vi "MQTT_Read_Subscribed_Topics.vi"(8 "error in (no error)":errorcluster) -> (0 "error out":errorcluster)   [LabVIEW 2020, in "MQTT_Functions.lvlib"]
doc: "A basic example that reads topics that the client subcribed to. \n\n© 2015 - daq.io, LLC - Peter Adelhardt"
uses:
  MQTT_Functions.lvlib
  Controls/QoS.ctl
  Controls/Connect_Flags.ctl
  Controls/Retain_Flag.ctl
  Controls/DUP_Flag.ctl
  Controls/User_Info.ctl
  Controls/Connection_Return_Codes.ctl
panel:
  out "Connection Status":T1=enum."Connection refused: not authorized"
  in  "Exit":bool
  in  "MQTT Broker":cluster{"address (IP)":string, "port":u16}={"address (IP)"="172.16.0.250", "port"=1883}
  out "Message IDs":u16[](array[numeric]) format="%x"
  out "Topics":string[](array[string])
  out "Messages":string[](array[string])
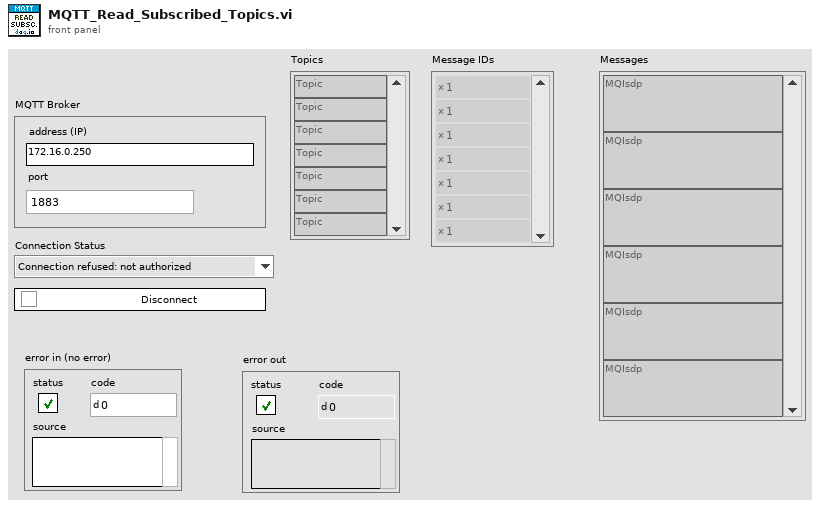
[diagram p1: front panel]
types:
  T1 = typedef "MQTT_Functions.lvlib/Connection_Return_Codes.ctl" = enum16{"Connection accepted", "Connection refused: unacceptable protocol version", "Connection refused: identifier rejected", "Connection refused: Server unavailable", "Connection refused: bad user name or password", "Connection refused: not authorized"}
  T2 = typedef "MQTT_Functions.lvlib/User_Info.ctl" = cluster{"User Name":string, "Password":string}
  T3 = typedef "MQTT_Functions.lvlib/QoS.ctl" = enum8{"At most once", "At least once", "Exactly once", "Reserved"}
  T4 = typedef "MQTT_Functions.lvlib/DUP_Flag.ctl" = bool
  T5 = typedef "MQTT_Functions.lvlib/Retain_Flag.ctl" = bool
  T6 = cluster{"QoS":T3, "DUP":T4, "Retain":T5, "Keep Alive (sec)":u16}
  T7 = typedef "MQTT_Functions.lvlib/Connect_Flags.ctl" = cluster{"user name":bool, "password":bool, "will retain":bool, "will flag":bool, "clean session":bool, "reserved":bool, "will QoS":T3}
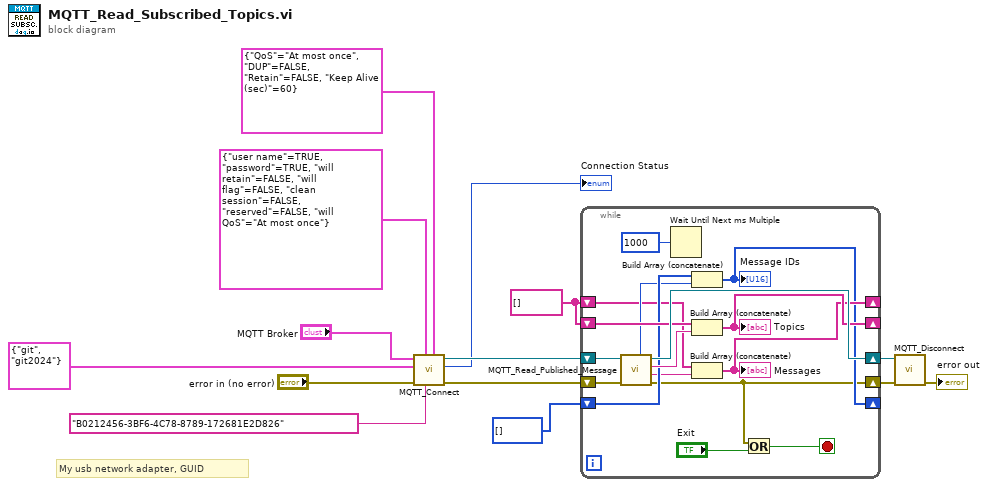
[diagram p0: block diagram]
diagram:
  w7 = string[] []
  # "My usb network adapter, GUID"
  n1 = call "MQTT_Connect.vi"("Connect Meta"=T6 {"QoS"=enum."At most once", "DUP"=FALSE, "Retain"=FALSE, "Keep Alive (sec)"=60}, "Client ID"="B0212456-3BF6-4C78-8789-172681E2D826", "Connect Flags"=T7 {"user name"=TRUE, "password"=TRUE, "will retain"=FALSE, "will flag"=FALSE, "clean session"=FALSE, "reserved"=FALSE, "will QoS"=enum."At most once"}, "error in (no error)"="error in (no error)", "User Info"=T2 {"User Name"="git", "Password"="git2024"}, "MQTT Broker"="MQTT Broker") -> ("error out"=w2:errorcluster, "Connection Status"=→"Connection Status":T1, "connection ID out"=w4:refnum<k5>)  [unwired: 3 in]
  n2 = while {
    shift-right: [w15] -> w9
    shift-left: w2 -> [w27]
    shift-right: [w17] -> _
    shift-left: u16[] [] -> [w23]
    shift-right: [w18] -> _
    shift-left: w7 -> [w21]
    shift-right: [w19] -> _
    shift-left: w7 -> [w25]
    shift-right: [w26] -> w10
    shift-left: w4 -> [w28]
    stop <- w16 stop-if-true
    n3 = call "MQTT_Read_Published_Message.vi"("error in (no error)"=w27, "connection ID"=w28) -> ("error out"=w15:errorcluster, "Message"=w20:string, "Topic Name"=w24:string, "connection ID out"=w26:refnum<k5>, "Message ID"=w22:u16)  [unwired: 4 in, 1 out]
    n4 = Wait Until Next ms Multiple(millisecond multiple=u32 1000) -> ()  [unwired: 1 out]
    n5 = Build Array (concatenate)(w23, w22) -> (w17:u16[])
    "Message IDs" <- w17
    n6 = Build Array (concatenate)(w25, w24) -> (w19:string[])
    "Topics" <- w19
    n7 = Build Array (concatenate)(w21, w20) -> (w18:string[])
    "Messages" <- w18
    n8 = Or(x=w15, y="Exit") -> (x .or. y?=w16:bool)
  }
  n9 = call "MQTT_Disconnect.vi"("error in (no error)"=w9, "connection ID"=w10) -> ("error out"=→"error out":errorcluster)  [unwired: 9 in]
